vi "IVI Error Converter.vi"(8 "error in (no error)":errorcluster {"code" format="%.0x"}, 10 "IVI error code (0)":i32 format="%.0x", 11 "instrument handle":u32) -> (0 "error out":errorcluster {"code" format="%.0x"}, 3 "instrument handle out":u32)   [LabVIEW 2009, in "Keysight XSAn.lvlib"]
doc: "This VI converts error codes from IVI instrument drivers to standard LabVIEW error codes. If an error is detected the VI builds the appropriate error cluster that is readable by one of the error handlers supplied with LabVIEW."
uses:
  <instrlib>/Keysight XSAn/Keysight XSAn.lvlib
  AgXSAn.dll
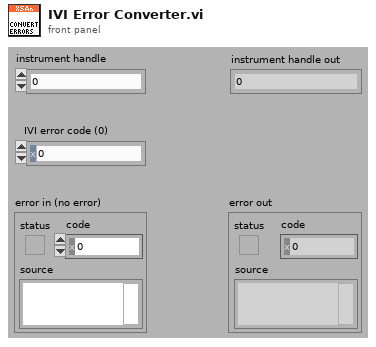
[diagram p1: front panel]
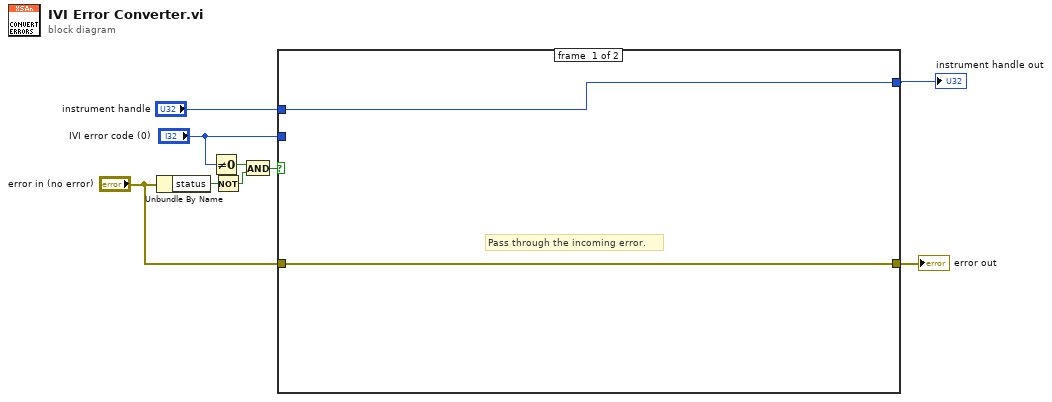
[diagram p0: block diagram]
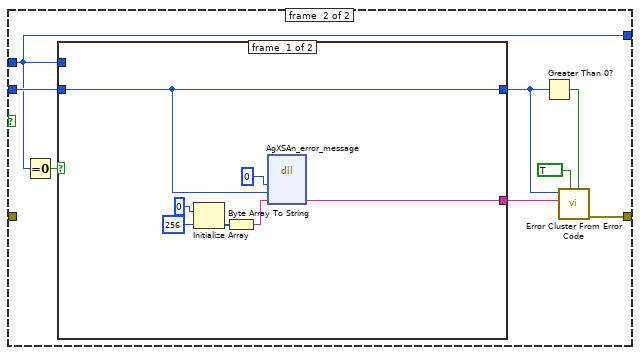
[diagram p2: hidden frame]
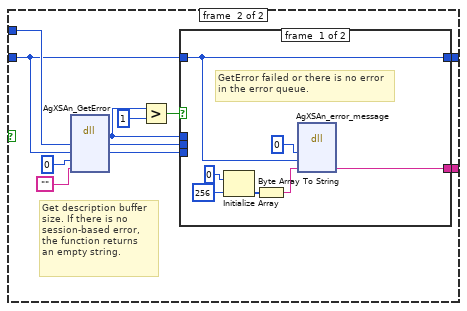
[diagram p3: hidden frame]
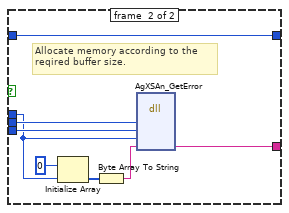
[diagram p4: hidden frame]
diagram:
  n1 = Unbundle By Name("error in (no error)") -> ("status"=w5:bool)
  n2 = Not Equal To 0?(x="IVI error code (0)") -> (x != 0?=w6:bool)
  n3 = Not(x=w5) -> (.not. x?=w4:bool)
  n4 = And(x=w6, y=w4) -> (x .and. y?=w3:bool)
  n5 = case shown="False" w3 {
    tunnel: "IVI error code (0)" -> [_ w19]
    tunnel: [w11 w14] -> w9
    tunnel: "instrument handle" -> [w10 w12]
    tunnel: "error in (no error)" -> [w11 _]
    tunnel: [w10 w12] -> w1
    frame #0 {
      # "Pass through the incoming error."
    }
    frame #1 {
      n6 = Equal To 0?(x=w12) -> (x = 0?=w13:bool)
      n7 = case shown="False" w13 {
        tunnel: w12 -> [_ w37]
        tunnel: w19 -> [w20 w29]
        tunnel: [w21 w28] -> w18
        tunnel: [w20 w27] -> w16
        frame #0 {
          n8 = Initialize Array(u8 0, 256) -> (w24:u8[])
          n9 = Byte Array To String(unsigned byte array=w24) -> (string=w26:string)
          n10 = dll-call lib="AgXSAn**.dll" fn="AgXSAn_error_message" label="error_message"("instrumentHandle"=0, "errorCode"=w20, "errorMessage"=w26) -> ("errorMessage"=w21:string)  [unwired: 5 in, 3 out]
        }
        frame #1 {
          # "Get description buffer\nsize. If there is no\nsession-based error,\nthe function returns\nan empty string."
          n11 = dll-call lib="AgXSAn**.dll" fn="AgXSAn_GetError" label="GetError"("vi"=w37, "errorCode"=w29, "bufferSize"=0, "description"="") -> ("return type"=w32:i32, "vi"=w31:u32, "errorCode"=w30:i32)  [unwired: 4 in, 3 out]
          n12 = Greater?(x=w32, y=1) -> (0:w33:bool)
          n13 = case shown="True" w33 {
            tunnel: w32 -> [_ w48]
            tunnel: w31 -> [_ w52]
            tunnel: w30 -> [_ w51]
            tunnel: [w38 w46] -> w28
            tunnel: w29 -> [w39 w45]
            tunnel: [w39 w45] -> w27
            frame #0 {
              # "GetError failed or there is no error\nin the error queue."
              n14 = Initialize Array(u8 0, 256) -> (w42:u8[])
              n15 = Byte Array To String(unsigned byte array=w42) -> (string=w44:string)
              n16 = dll-call lib="AgXSAn**.dll" fn="AgXSAn_error_message" label="error_message"("instrumentHandle"=0, "errorCode"=w39, "errorMessage"=w44) -> ("errorMessage"=w38:string)  [unwired: 5 in, 3 out]
            }
            frame #1 {
              # "Allocate memory according to the\nreqired buffer size."
              n17 = Initialize Array(u8 0, w48) -> (w50:u8[])
              n18 = Byte Array To String(unsigned byte array=w50) -> (string=w47:string)
              n19 = dll-call lib="AgXSAn**.dll" fn="AgXSAn_GetError" label="GetError"("vi"=w52, "errorCode"=w51, "bufferSize"=w48, "description"=w47) -> ("description"=w46:string)  [unwired: 6 in, 3 out]
            }
          }
        }
      }
      n20 = Greater Than 0?(x=w16) -> (x > 0?=w15:bool)
      n21 = call <vilib>:"Error Cluster From Error Code.vi"("is warning? (False)"=w15, "show call chain? (False)"=TRUE, "error message (\"\")"=w18, "error code (0)"=w16) -> ("error out"=w14:errorcluster)  [unwired: 1 in, 4 out]
    }
  }
  "error out" <- w9
  "instrument handle out" <- w1
